vi "Initialize-FilterWheel-SubVI.vi"() -> (7 "VISA resource name out":refnum<visa-resource-name>, 10 "error out":errorcluster)   [LabVIEW 2014]
uses:
  <vilib>/Instr/_visa.llb/VISA Configure Serial Port (Instr).vi
panel:
  in  "Serial port":refnum<visa-resource-name>="COM1"
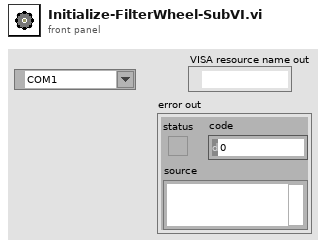
[diagram p1: front panel]
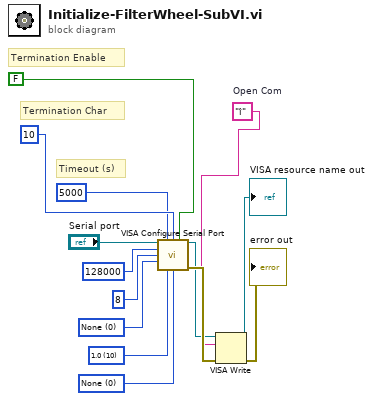
[diagram p0: block diagram]
diagram:
  w1 = "î"  # Open Com
  w6 = u16 0 items=["None"=0, "XON/XOFF"=1, "RTS/CTS"=2, "DTR/DSR"=4] ("flow control")
  w7 = u16 10 items=["1.0"=10, "1.5"=15, "2.0"=20] ("stop bits")
  w8 = u16 0 items=["None", "Odd", "Even", "Mark", "Space"] ("parity")
  # "Termination Char"
  # "Termination Enable"
  # "Timeout (s)"
  n1 = call-poly "VISA Configure Serial Port"("VISA resource name"="Serial port", "timeout (10sec)"=u32 5000 ("timeout (ms)"), "termination char\n(0xA = '\\n' = LF)"=u8 10 ("termination char\n(0xA = '\\n' = LF)"), "Enable Termination\nChar (T)"=FALSE ("End read on termination character?"), "baud rate (9600)"=u32 128000 ("timeout (ms)"), "data bits (8)"=u16 8 ("data bits"), "parity (0:none)"=w8, "stop bits (10: 1 bit)"=w7, "flow control (0:none)"=w6) -> ("VISA resource name out"=w4:refnum<visa-resource-name>, "error out"=w5:errorcluster)  [unwired: 5 in]
  n2 = VISA Write(VISA resource name=w4, write buffer=w1, error in (no error)=w5) -> (VISA resource name out=→"VISA resource name out":refnum<visa-resource-name>, error out=→"error out":errorcluster)  [unwired: 1 out]
